vi "ctrl-c.vi"(8 "error in (no error)":errorcluster, 11 "dotnet_system_exec in":refnum<class "dotnet_system_exec.lvclass">) -> (0 "error out":errorcluster, 3 "dotnet_system_exec out":refnum<class "dotnet_system_exec.lvclass">)   [LabVIEW 2020, in "dotnet_system_exec.lvclass"]
uses:
  dotnet_system_exec.lvclass
  dotnet_system_exec.lvclass/dotnet_system_exec.ctl
  KERNEL32.DLL
  bb9f7f1a-5c89-45c4-ba54-91e94f581c16.vi
  9ea30695-a94b-45f7-a525-b363fb18392c.vi
  06c012ef-9450-451d-a724-8edd82485dc0.vi
  c05b488f-5d94-4582-b0b6-f445098539e1.vi
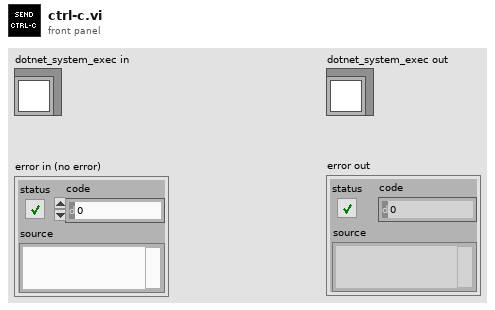
[diagram p1: front panel]
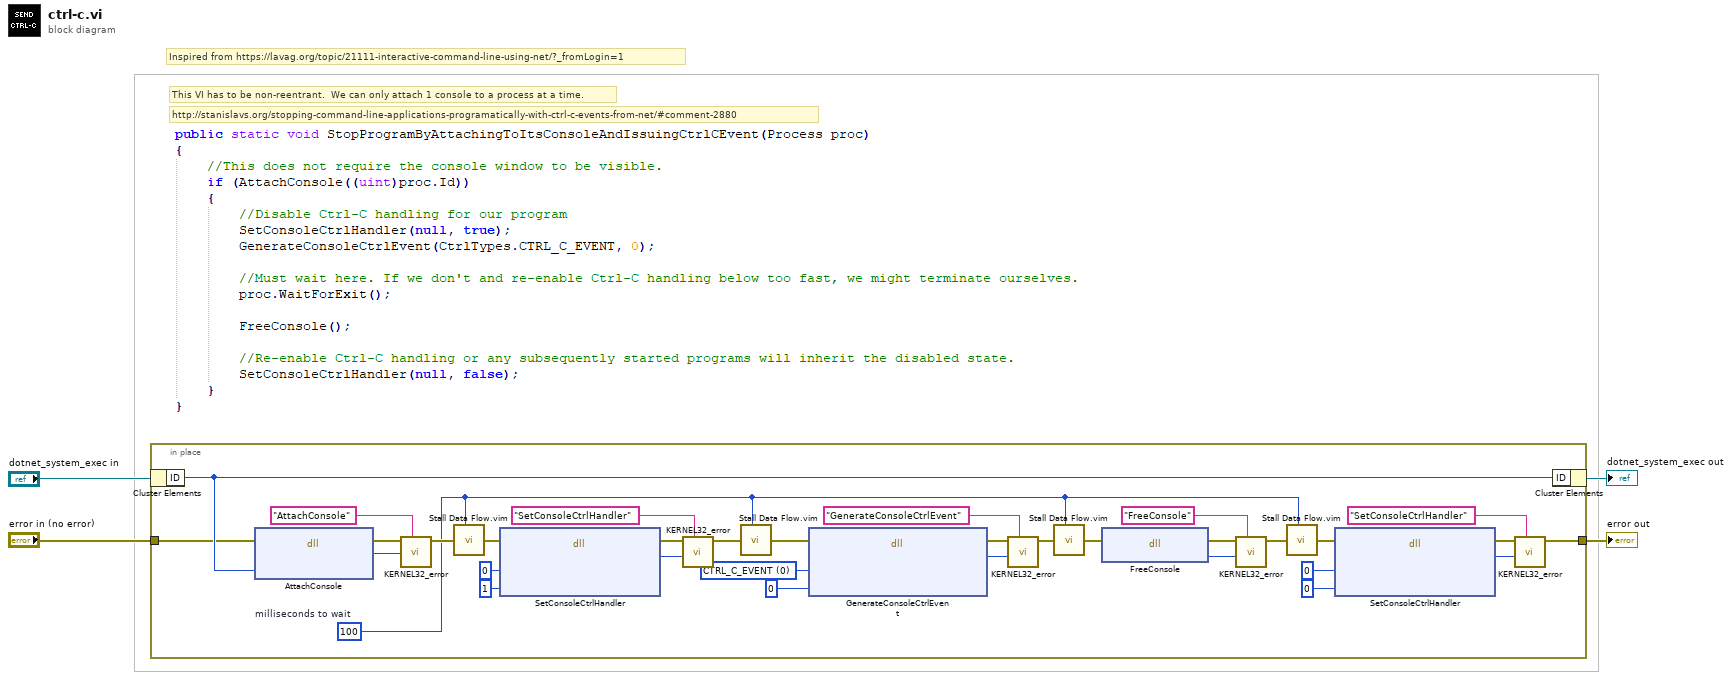
[diagram p0: block diagram]
diagram:
  # "Inspired from https://lavag.org/topic/21111-interactive-command-line-using-net/?_fromLogin=1"
  # "This VI has to be non-reentrant.  We can only attach 1 console to a process at a time."
  # "http://stanislavs.org/stopping-command-line-applications-programatically-with-ctrl-c-events-from-net/#comment-2880"
  n1 = in-place {
    in-place-border: [w10] -> w3
    in-place-border: "error in (no error)" -> [w35]
    w5 = u32 100  # milliseconds to wait
    w34 = 0 items=["CTRL_C_EVENT", "CTRL_BREAK_EVENT"]
    n2 = in-place-cluster #1("dotnet_system_exec in") -> ("ID"=w36:i32)
    n3 = dll-call lib="KERNEL32.DLL" fn="AttachConsole" ("GetSystemPowerStatus")(error in=w35, "dwProcessId"=w36) -> (error out=w29:errorcluster, "return type"=w27:i32)  [unwired: 2 in, 2 out]
    n4 = call "KERNEL32_error.vi"("name"="AttachConsole", "return"=w27, "error in (no error)"=w29) -> ("error out"=w28:errorcluster)  [unwired: 8 in]
    n5 = call "Stall Data Flow.vim"("value in"=w28, "milliseconds to wait"=w5) -> ("value out"=w9:errorcluster)  [unwired: 1 out]
    n6 = dll-call lib="KERNEL32.DLL" fn="SetConsoleCtrlHandler" ("GetSystemPowerStatus")(error in=w9, "HandlerRoutine"=0, "Add"=1) -> (error out=w25:errorcluster, "return type"=w24:i32)  [unwired: 2 in, 3 out]
    n7 = call "KERNEL32_error.vi"("name"="SetConsoleCtrlHandler", "return"=w24, "error in (no error)"=w25) -> ("error out"=w22:errorcluster)  [unwired: 8 in]
    n8 = call "Stall Data Flow.vim"("value in"=w22, "milliseconds to wait"=w5) -> ("value out"=w8:errorcluster)  [unwired: 1 out]
    n9 = dll-call lib="KERNEL32.DLL" fn="GenerateConsoleCtrlEvent" ("GetSystemPowerStatus")(error in=w8, "dwCtrlEvent"=w34, "dwProcessGroupId"=0 ("dwCtrlEvent")) -> (error out=w21:errorcluster, "return type"=w20:i32)  [unwired: 2 in, 3 out]
    n10 = call "KERNEL32_error.vi"("name"="GenerateConsoleCtrlEvent", "return"=w20, "error in (no error)"=w21) -> ("error out"=w18:errorcluster)  [unwired: 8 in]
    n11 = call "Stall Data Flow.vim"("value in"=w18, "milliseconds to wait"=w5) -> ("value out"=w7:errorcluster)  [unwired: 1 out]
    n12 = dll-call lib="KERNEL32.DLL" fn="FreeConsole" ("GetSystemPowerStatus")(error in=w7) -> (error out=w17:errorcluster, "return type"=w16:i32)  [unwired: 2 in, 1 out]
    n13 = call "KERNEL32_error.vi"("name"="FreeConsole", "return"=w16, "error in (no error)"=w17) -> ("error out"=w14:errorcluster)  [unwired: 8 in]
    n14 = call "Stall Data Flow.vim"("value in"=w14, "milliseconds to wait"=w5) -> ("value out"=w6:errorcluster)  [unwired: 1 out]
    n15 = dll-call lib="KERNEL32.DLL" fn="SetConsoleCtrlHandler" ("GetSystemPowerStatus")(error in=w6, "HandlerRoutine"=0, "Add"=0) -> (error out=w13:errorcluster, "return type"=w12:i32)  [unwired: 2 in, 3 out]
    n16 = call "KERNEL32_error.vi"("name"="SetConsoleCtrlHandler", "return"=w12, "error in (no error)"=w13) -> ("error out"=w10:errorcluster)  [unwired: 8 in]
    n17 = in-place-cluster #1("ID"=w36) -> (→"dotnet_system_exec out":refnum<class "dotnet_system_exec.lvclass">)
  }
  "error out" <- w3
